vi "Body References FGV.vi"(6 "Destroy References?":bool=TRUE, 8 "error in (no error)":errorcluster, 11 "BodyData":T1) -> (0 "error out":errorcluster)   [LabVIEW 2014]
uses:
  Type Defs/BodyData.ctl
  Type Defs/ClippedEdges.ctl
  Type Defs/HandLeftConfidence.ctl
  Type Defs/HandLeftState.ctl
  Type Defs/HandRightConfidence.ctl
  Type Defs/HandRightState.ctl
  Microsoft.Kinect
  Type Defs/LeanTrackingState.ctl
  LVH-KinectOne.lvlib
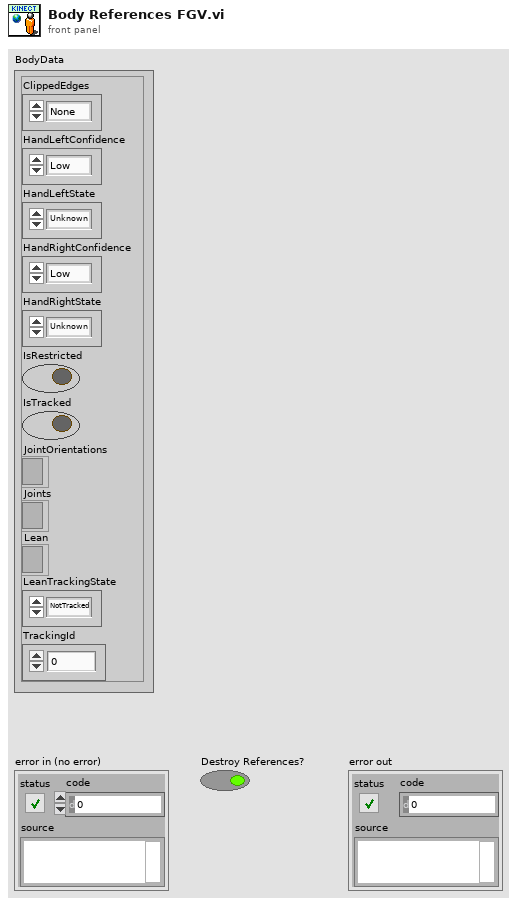
[diagram p1: front panel]
types:
  T1 = typedef "LVH-KinectOne.lvlib/BodyData.ctl" = cluster{"ClippedEdges":T2, "HandLeftConfidence":T3, "HandLeftState":T4, "HandRightConfidence":T5, "HandRightState":T6, "IsRestricted":bool, "IsTracked":bool, "JointOrientations":refnum<k24>, "Joints":refnum<k24>, "Lean":refnum<k24>, "LeanTrackingState":T7, "TrackingId":u64}
  T2 = typedef "LVH-KinectOne.lvlib/ClippedEdges.ctl" = enum16{"None", "Right", "Left", "Top", "Bottom"}
  T3 = typedef "LVH-KinectOne.lvlib/HandLeftConfidence.ctl" = enum16{"Low", "High"}
  T4 = typedef "LVH-KinectOne.lvlib/HandLeftState.ctl" = enum16{"Unknown", "NotTracked", "Open", "Closed", "Lasso"}
  T5 = typedef "LVH-KinectOne.lvlib/HandRightConfidence.ctl" = enum16{"Low", "High"}
  T6 = typedef "LVH-KinectOne.lvlib/HandRightState.ctl" = enum16{"Unknown", "NotTracked", "Open", "Closed", "Lasso"}
  T7 = typedef "LVH-KinectOne.lvlib/LeanTrackingState.ctl" = enum16{"NotTracked", "Inferred", "Tracked"}
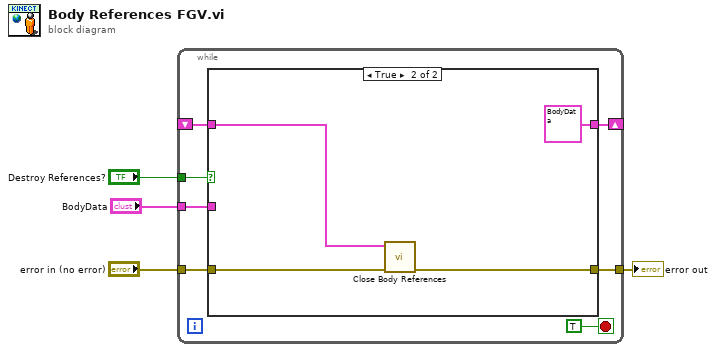
[diagram p0: block diagram]
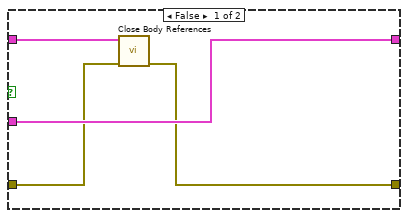
[diagram p2: hidden frame]
diagram:
  n1 = while {
    tunnel: "BodyData" -> [w10]
    shift-right: [w9] -> _
    shift-left: _ -> [w8]
    tunnel: "error in (no error)" -> [w7]
    tunnel: [w6] -> w1
    tunnel: "Destroy References?" -> [w5]
    stop <- TRUE stop-if-true
    n2 = case shown="True" w5 {
      tunnel: w10 -> [w15 _]
      tunnel: [w15 T1 {"ClippedEdges"=enum."None", "HandLeftConfidence"=enum."Low", "HandLeftState"=enum."Unknown", "HandRightConfidence"=enum."Low", "HandRightState"=enum."Unknown", "IsRestricted"=FALSE, "IsTracked"=FALSE, "JointOrientations"=refnum, "Joints"=refnum, "Lean"=refnum, "LeanTrackingState"=enum."NotTracked", "TrackingId"=0} ("BodyData")] -> w9
      tunnel: w8 -> [w14 w18]
      tunnel: w7 -> [w13 w19]
      tunnel: [w12 w16] -> w6
      frame False {
        n3 = call "Close Body References.vi"("Error In"=w13, "BodyData"=w14) -> ("Error Out"=w12:errorcluster)  [unwired: 9 in]
      }
      frame True {
        n4 = call "Close Body References.vi"("Error In"=w19, "BodyData"=w18) -> ("Error Out"=w16:errorcluster)  [unwired: 9 in]
      }
    }
  }
  "error out" <- w1
